vi "Send S&E EVENT message.vi"(1 "Event Source(user)":T1, 2 "Send(T)":bool=TRUE, 5 "Source Info(no info)":string, 7 "Event Description":string, 9 "error in (no error)":errorcluster, 12 "Loc Sub ID/Event ID(No ID)":u16=9999, 13 "Elevated priority":bool) -> (6 "Loop ID out":u16, 10 "error out":errorcluster)   [LabVIEW 2011]
doc: "Put error message in the S&E Q. CAn also send if no error, debends exclusively on boolean in."
uses:
  S&E Event source.ctl
  emi Lib/System 01/0 - General/S&E reporting/Private/_emi_ S&E Message.ctl
  emi Lib/System 01/0 - General/S&E reporting/Private/_emi_ S&E Message type.ctl
  S&E Event Type.ctl
  emi Lib/System 01/0 - General/Private/_emi_GFV System ID.vi
panel:
  in  "Loop ID in(No Loop)":u16=9999
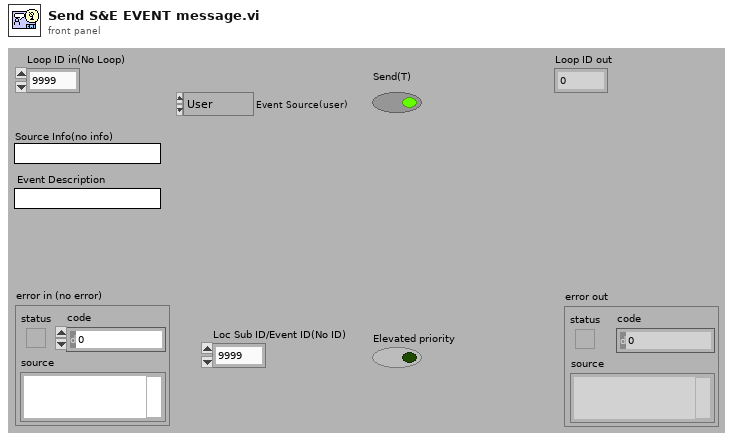
[diagram p1: front panel]
types:
  T1 = typedef "S&E Event source.ctl" = enum16{"User", "Instrument", "Application", "Windows"}
  T2 = typedef "S&E Event Type.ctl" = cluster{"Event Source":T1, "Source Info":string, "Event Description":string}
  T3 = typedef "_emi_ S&E Message type.ctl" = enum16{"Error/Warning", "Note", "Debug", "Event", "Alarm Analog", "Alarm Digital", "Annotation"}
  T4 = typedef "_emi_ S&E Message.ctl" = cluster{"Type":T3, "Originate time":dbl, "System":u8, "Loop":u16, "Sub ID":u16, "Elevated priority":bool, "E&S Message content":variant}
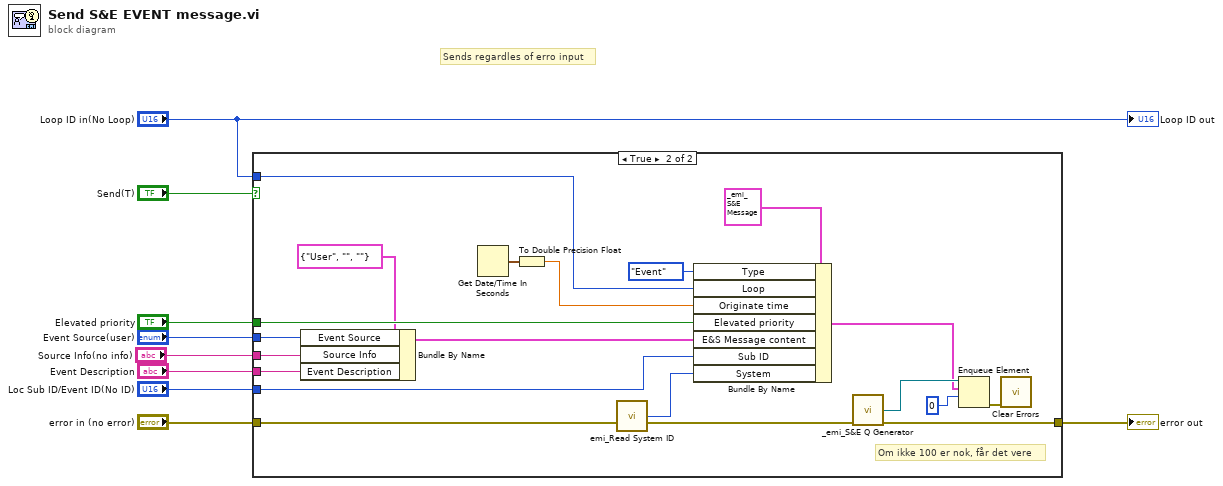
[diagram p0: block diagram]
diagram:
  # "Sends regardles of erro input"
  n1 = case shown="True" "Send(T)" {
    tunnel: "Loop ID in(No Loop)" -> [_ w26]
    tunnel: "Elevated priority" -> [_ w27]
    tunnel: "error in (no error)" -> [w10 w18]
    tunnel: [w10 w24] -> w6
    tunnel: "Loc Sub ID/Event ID(No ID)" -> [_ w20]
    tunnel: "Event Source(user)" -> [_ w13]
    tunnel: "Event Description" -> [_ w12]
    tunnel: "Source Info(no info)" -> [_ w11]
    frame False {
    }
    frame True {
      # "Om ikke 100 er nok, får det vere"
      n2 = Bundle By Name(cluster=T2 {"Event Source"=enum."User", "Source Info"="", "Event Description"=""} ("S&E Event"), "Event Source"=w13, "Source Info"=w11, "Event Description"=w12) -> (w14:T2)
      n3 = Get Date/Time In Seconds() -> (seconds since 1Jan1904=w28:timestamp)
      n4 = To Double Precision Float(number=w28) -> (double precision float=w29:dbl)
      n5 = call "emi_Read System ID.vi"("error in (no error)"=w18) -> ("System ID"=w16:u8, "error out"=w17:errorcluster)  [unwired: 13 in]
      n6 = Bundle By Name(cluster=T4 {"Type"=enum."Error/Warning", "Originate time"=0.0, "System"=0, "Loop"=0, "Sub ID"=0, "Elevated priority"=FALSE, "E&S Message content"=variant} ("E&S Message"), "Type"=_emi__S&E_Message_type."Event", "Loop"=w26, "Originate time"=w29, "Elevated priority"=w27, "E&S Message content"=w14, "Sub ID"=w20, "System"=w16) -> (w22:T4)
      n7 = call "_emi_S&E Q Generator.vi"("error in (no error)"=w17) -> ("E&S Message Q"=w23:refnum<queue>, "error out"=w24:errorcluster)  [unwired: 13 in]
      n8 = Enqueue Element(queue=w23, element=w22, timeout in ms (-1)=0) -> (error out=w19:errorcluster)  [unwired: 1 in, 2 out]
      n9 = call <vilib>:"Clear Errors.vi"("error in (no error)"=w19) -> ()  [unwired: 6 in, 1 out]
    }
  }
  "error out" <- w6
  "Loop ID out" <- "Loop ID in(No Loop)"
